vi "Read Alicat Data.vi"(8 "error in (no error)":errorcluster, 11 "Nicholas Data in":refnum<class "Nicholas Data.lvclass">) -> (0 "error out":errorcluster, 2 "Alicat Data":refnum<class "Alicat Data.lvclass">[](array[class]), 3 "Nicholas Data out":refnum<class "Nicholas Data.lvclass">)   [LabVIEW 2016, in "Nicholas Data.lvclass"]
uses:
  Nicholas Data.lvclass
  <vilib>/MSR Consulting, LLC/Devices/Alicats/Data/Alicat Data.lvclass
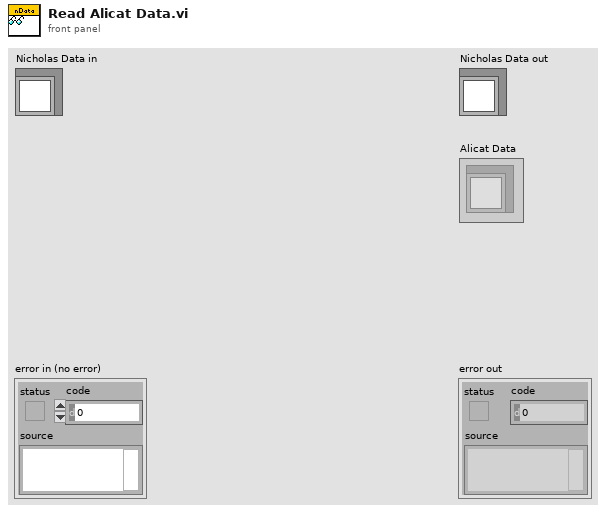
[diagram p1: front panel]
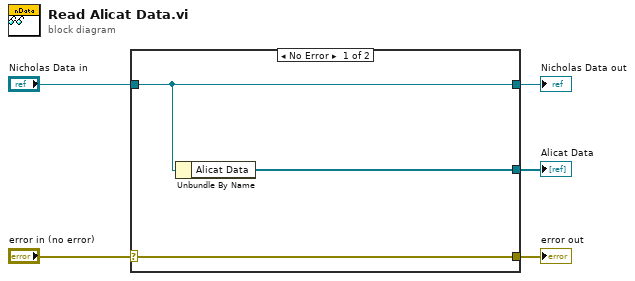
[diagram p0: block diagram]
diagram:
  n1 = case shown="No Error" "error in (no error)" {
    selector: "error in (no error)" -> [w8 w9]
    tunnel: [w8 w9] -> w4
    tunnel: [w7 w10] -> w2
    tunnel: "Nicholas Data in" -> [w7 w10]
    tunnel: [w6 _] -> w1
    frame No Error {
      n2 = Unbundle By Name(w7) -> ("Alicat Data"=w6:refnum<class "Alicat Data.lvclass">[])
    }
    frame Error {
    }
  }
  "error out" <- w4
  "Nicholas Data out" <- w2
  "Alicat Data" <- w1
